vi "Resource from String.vi"(8 "error in (no error)":errorcluster, 10 "Resource from String":string, 11 "Generic Controller in":refnum<class "Generic Plugin.lvclass">) -> (0 "error out":errorcluster, 2 "Resource as Variant":variant, 3 "Generic Controller out":refnum<class "Generic Plugin.lvclass">)   [LabVIEW 2020, in "Generic Plugin.lvclass"]
uses:
  Generic Plugin.lvclass
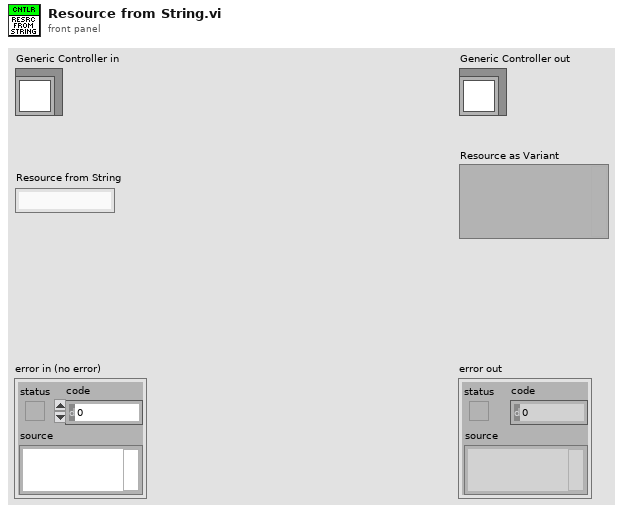
[diagram p1: front panel]
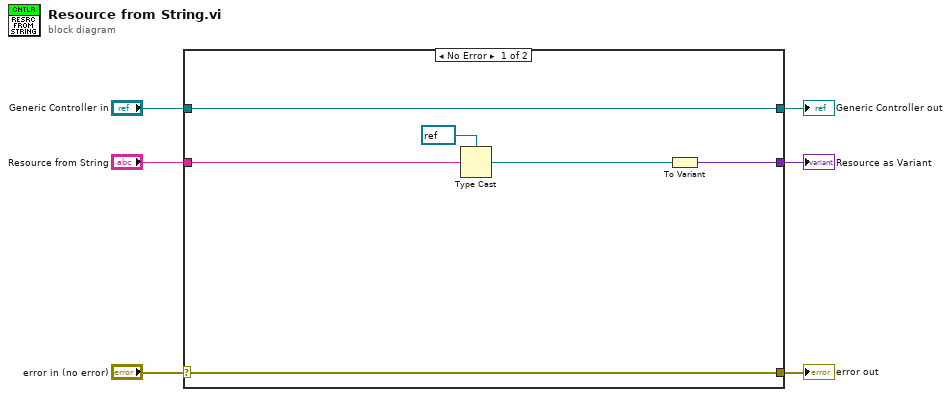
[diagram p0: block diagram]
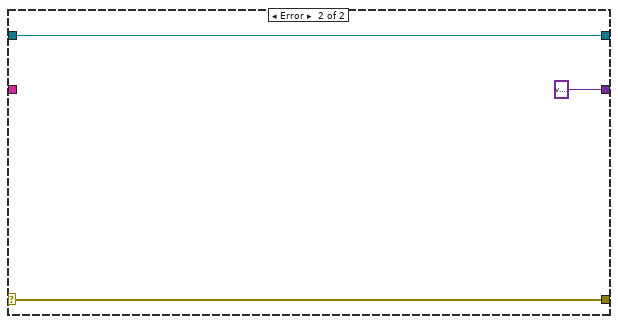
[diagram p2: hidden frame]
diagram:
  n1 = case shown="No Error" "error in (no error)" {
    selector: "error in (no error)" -> [w11 w15]
    tunnel: [w11 w15] -> w5
    tunnel: [w12 w14] -> w3
    tunnel: "Generic Controller in" -> [w12 w14]
    tunnel: "Resource from String" -> [w10 _]
    tunnel: [w8 variant ("Resource as Variant")] -> w1
    frame No Error {
      n2 = Type Cast(type=refnum<visa-resource-name> refnum ("VISA resource name"), x=w10) -> (*(type *) &x=w9:refnum<visa-resource-name>)
      n3 = To Variant(anything=w9) -> (Variant=w8:variant)
    }
    frame Error {
    }
  }
  "error out" <- w5
  "Generic Controller out" <- w3
  "Resource as Variant" <- w1
